vi "Get SMO Name.vi"(8 "error in (no error)":errorcluster, 11 "instrument.PPMS2 in":refnum<class "instrument.PPMS2.lvclass">) -> (0 "error out":errorcluster, 2 "SMO Name":string, 3 "instrument.PPMS2 out":refnum<class "instrument.PPMS2.lvclass">)   [LabVIEW 2019, in "instrument.PPMS2.lvclass"]
uses:
  instrument.PPMS2.lvclass
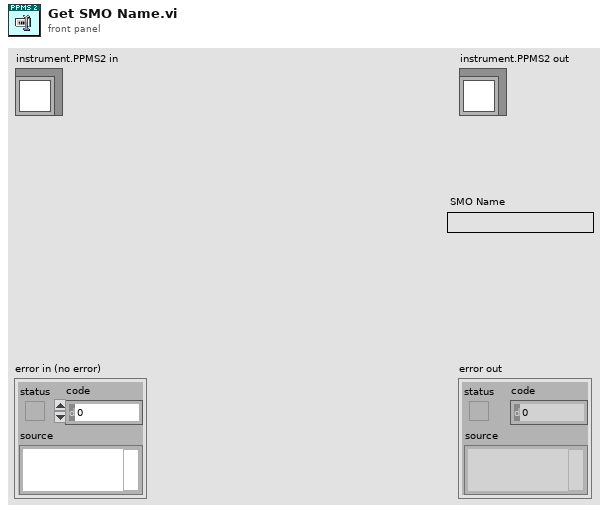
[diagram p1: front panel]
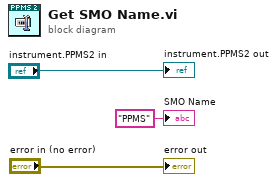
[diagram p0: block diagram]
diagram:
  "error out" <- "error in (no error)"
  "instrument.PPMS2 out" <- "instrument.PPMS2 in"
  "SMO Name" <- "PPMS" ("SMO Name")
